vi "Large current measurement readings.vi"() -> ()   [LabVIEW 2016, in "Top Level.lvlib"]
doc: "This vi displays current measurements in a large format"
uses:
  Top Level.lvlib
  Controls/Vertical Rod states.ctl
panel:
  in  "Tab Control":enum32{"measurements", "error and scale factor"}(tab)
  out "Cathode on":bool
  in  "rare count rate or stable":bool
  out "injector current":dbl format="%.2p"
  out "Current measurements":dbl(graph)
  out "offset cup Actual":dbl format="%#_5g"
  out "Current":dbl format="%#_4p"
  in  "stop":bool
  in  "error in (no error)":errorcluster
  out "error out":errorcluster
  out "Numeric":i32
  # "Rare count rate"
  # "Stable current"
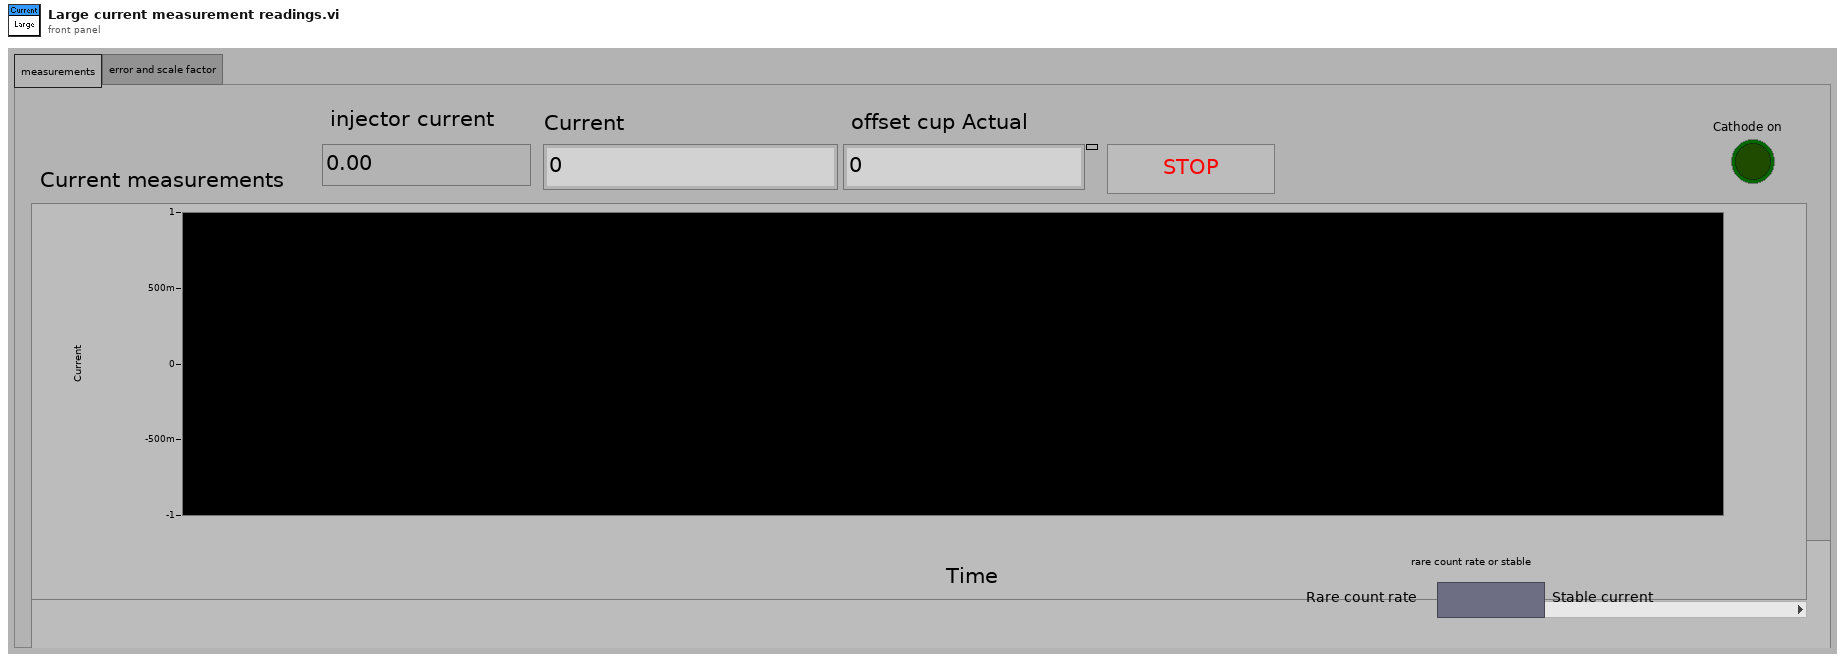
[diagram p1: front panel]
types:
  T1 = typedef "Vertical Rod states.ctl" = enum16{"status unclear", "rod down", "rod up"}
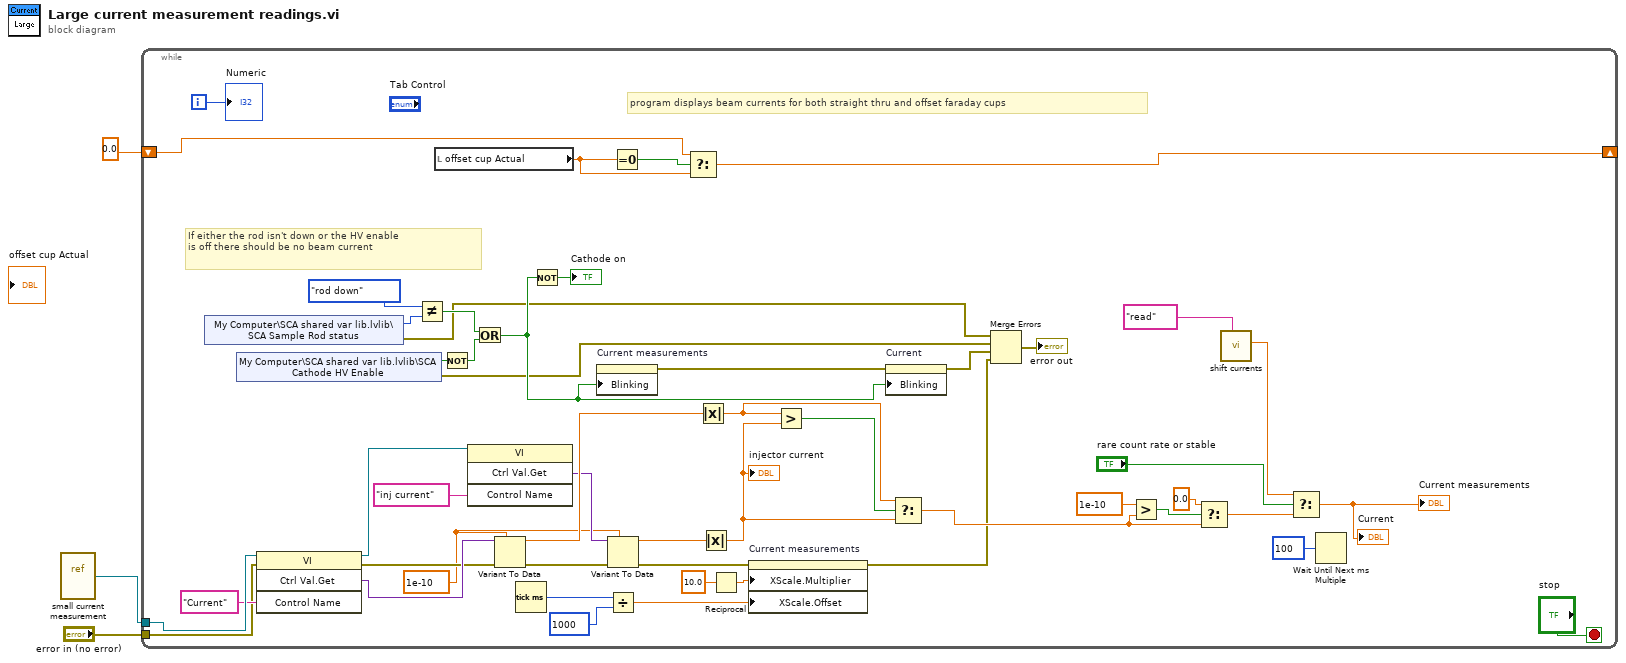
[diagram p0: block diagram]
diagram:
  n1 = vi-ref "small current measurement.vi"() -> (w2:refnum<vi>)
  n2 = while {
    shift-right: [w45] -> _
    shift-left: 0.0 -> [w46]
    tunnel: "error in (no error)" -> [w41]
    tunnel: w2 -> [w43]
    i -> [w38]
    stop <- "stop" stop-if-true
    w26 = 1e-10 ("x")
    # "If either the rod isn't down or the HV enable\nis off there should be no beam current"
    # "program displays beam currents for both straight thru and offset faraday cups"
    n3 = shared-variable "My Computer\\SCA shared var lib.lvlib\\SCA Sample Rod status"() -> (w15:T1, error out=w6:errorcluster)  [unwired: 1 in]
    n4 = shared-variable "My Computer\\SCA shared var lib.lvlib\\SCA Cathode HV Enable"() -> (w13:bool, error out=w7:errorcluster)  [unwired: 1 in]
    n5 = invoke class="VI" method="Ctrl Val.Get"(reference=w43, error in=w41, "Control Name"="Current") -> (reference out=w29:refnum<vi>, error out=w36:errorcluster, "Get Control Value Variant"=w40:variant)  [unwired: 1 in, 1 out]
    n6 = Not Equal?(x=Vertical_Rod_states."rod down", y=w15) -> (x != y?=w11:bool)
    n7 = local read "offset cup Actual"() -> (w37:dbl)
    n8 = Not(x=w13) -> (.not. x?=w12:bool)
    n9 = invoke class="VI" method="Ctrl Val.Get"(reference=w29, "Control Name"="inj current") -> ("Get Control Value Variant"=w27:variant)  [unwired: 2 in, 3 out]
    n10 = Or(x=w11, y=w12) -> (x .or. y?=w10:bool)
    n11 = Variant To Data(error in=w36, type=w26, Variant=w40) -> (data=w39:dbl, error out=w25:errorcluster)
    n12 = Tick Count (ms)() -> (millisecond timer value=w16:u32)
    n13 = Not(x=w10) -> (.not. x?=→"Cathode on":bool)
    n14 = property on="Current measurements" class="WFChart (strict)"("Blinking"=w10) -> (error out=w30:errorcluster)  [unwired: 2 in, 1 out]
    n15 = Variant To Data(error in=w25, type=w26, Variant=w27) -> (data=w24:dbl, error out=w19:errorcluster)
    n16 = Divide(x=w16, y=u32 1000 ("x")) -> (x/y=w18:dbl)
    n17 = Equal To 0?(x=w37) -> (x = 0?=w47:bool)
    n18 = Select(t=w46, s=w47, f=w37) -> (s? t:f=w45:dbl)
    n19 = Absolute Value(x=w39) -> (abs(x)=w44:dbl)
    n20 = Absolute Value(x=w24) -> (abs(x)=w23:dbl)
    "injector current" <- w23
    n21 = Reciprocal(x=10.0) -> (1/x=w21:dbl)
    n22 = property on="Current measurements" class="WFChart (strict)"(error in=w19, "XScale.Multiplier"=w21, "XScale.Offset"=w18) -> (error out=w9:errorcluster)  [unwired: 1 in, 1 out]
    n23 = Greater?(x=w44, y=w23) -> (0:w48:bool)
    n24 = property on="Current" class="DigNum (strict)"(error in=w30, "Blinking"=w10) -> (error out=w8:errorcluster)  [unwired: 1 in, 1 out]
    n25 = Select(t=w44, s=w48, f=w23) -> (s? t:f=w34:dbl)
    n26 = Merge Errors(w6, w7, w8, w9) -> (→"error out":errorcluster)
    n27 = Greater?(x=1e-10, y=w34) -> (0:w50:bool)
    n28 = Select(t=0.0, s=w50, f=w34) -> (s? t:f=w31:dbl)
    n29 = call "shift currents.vi"("Combo Box"="read") -> ("current out"=w32:dbl)  [unwired: 10 in]
    n30 = Select(t=w32, s="rare count rate or stable", f=w31) -> (s? t:f=→"Current" →"Current measurements":dbl)
    n31 = Wait Until Next ms Multiple(millisecond multiple=u32 100) -> ()  [unwired: 1 out]
    "Numeric" <- w38
  }
